vi "ReduceToConnectedAxes.vi"(8 "Axes à déplacer input":bool[](array[boolean]), 9 "Déplacements input":dbl[](array[numeric]), 10 "Axes connectés":string[](array[string])) -> (0 "Axes à déplacer output":bool[](array[boolean]), 1 "Déplacements output":dbl[](array[numeric]))   [LabVIEW 2013]
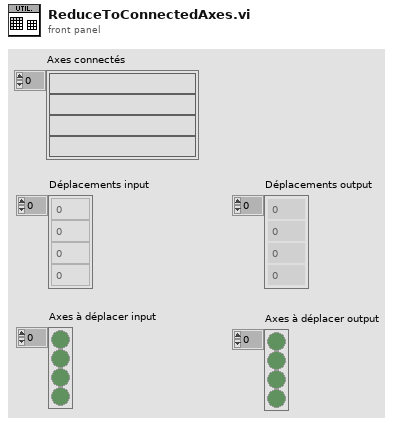
[diagram p1: front panel]
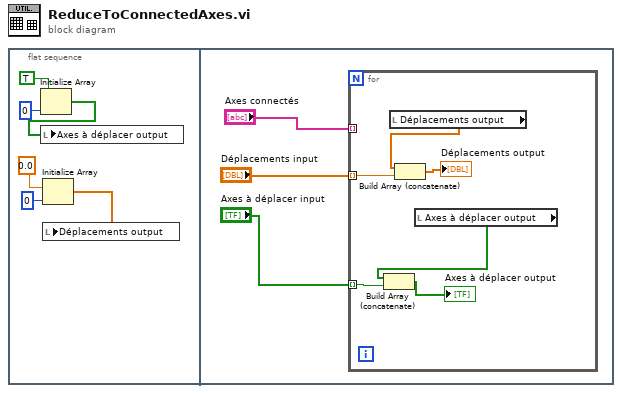
[diagram p0: block diagram]
diagram:
  n1 = flat-sequence {
    frame #0 {
      n2 = Initialize Array(TRUE, 0 ("taille de la dimension")) -> (w6:bool[])
      n3 = local write "Axes à déplacer output"(w6) -> ()
      n4 = Initialize Array(0.0, 0 ("taille de la dimension")) -> (w3:dbl[])
      n5 = local write "Déplacements output"(w3) -> ()
    }
    frame #1 {
      n6 = for {
        tunnel: "Axes connectés" -> [_] mode=indexing
        tunnel: "Déplacements input" -> [w15] mode=indexing
        tunnel: "Axes à déplacer input" -> [w13] mode=indexing
        n7 = local read "Déplacements output"() -> (w11:dbl[])
        n8 = Build Array (concatenate)(w11, w15) -> (→"Déplacements output":dbl[])
        n9 = local read "Axes à déplacer output"() -> (w10:bool[])
        n10 = Build Array (concatenate)(w10, w13) -> (→"Axes à déplacer output":bool[])
      }
    }
  }
